vi "New Parameter File.vi"(8 "error in":errorcluster) -> (0 "error out":errorcluster, 3 "new parameter file":refnum<k24>)   [LabVIEW 2020, in "AIM_Parameter_ni.lvlib"]
uses:
  AIM_Parameter_ni.lvlib
  C:/Users/Administrator/Desktop/GIT/Ballard-Arinc-429-XML-Generator/Source/Assemblies/Aim_Parameter_ni/bin/Debug/AIM_429_Parameter_ni.dll
  Assemblies/Aim_Parameter_ni/bin/Debug/AIM_429_Parameter_ni.dll
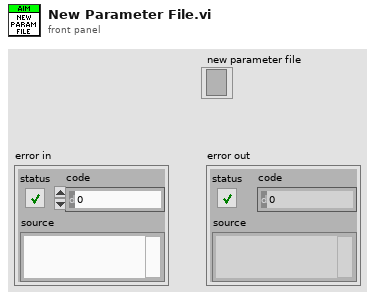
[diagram p1: front panel]
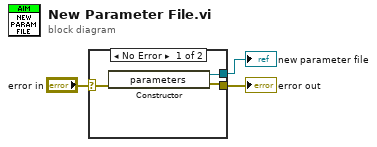
[diagram p0: block diagram]
diagram:
  n1 = case shown="No Error" "error in" {
    selector: "error in" -> [w6 _]
    tunnel: [w4 _] -> w1
    tunnel: [w5 _] -> w3
    frame No Error {
      n2 = constructor class="parameters"(error in=w6) -> (reference out=w4:refnum<k24>, error out=w5:errorcluster)  [unwired: 2 in, 1 out]
    }
    frame Error {
    }
  }
  "new parameter file" <- w1
  "error out" <- w3
